vi "RepIntCalc.vi"(8 "SpindleSize":i32, 9 "Look Ahead":i32, 10 "Interrupt Rate":i32=32, 11 "Current Encoder Position":i32) -> (3 "Diff Index":dbl)   [LabVIEW 2010, in "KevLib01.lvlib"]
uses:
  KevLib01.lvlib
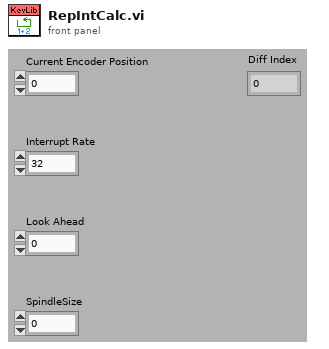
[diagram p1: front panel]
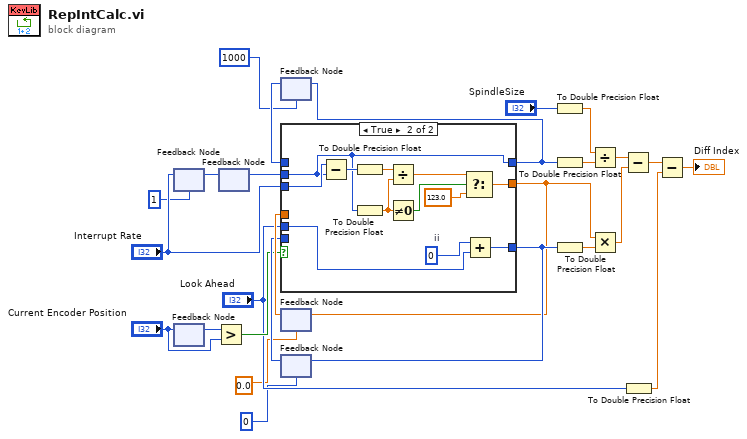
[diagram p0: block diagram]
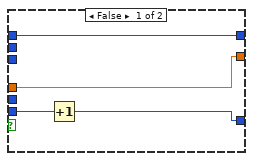
[diagram p2: hidden frame]
diagram:
  n1 = feedback-in #1("Interrupt Rate") -> ()
  n2 = feedback #1(1 ("Interrupt Rate")) -> (w2:i32)
  n3 = feedback-in #2("Current Encoder Position") -> ()
  n4 = feedback #2() -> (w20:i32)  [unwired: 1 out]
  n5 = Greater?(x=w20, y="Current Encoder Position") -> (0:w14:bool)
  n6 = feedback-in #3(w2) -> ()
  n7 = feedback #3() -> (w1:i32)  [unwired: 1 out]
  n8 = feedback #4(1000 ("Interrupt Rate")) -> (w24:i32)
  n9 = feedback #5(0.0 ("f")) -> (w16:dbl)
  n10 = feedback #6(0) -> (w15:i32)
  n11 = case shown="True" w14 {
    tunnel: [w29 w34] -> w19
    tunnel: w15 -> [w30 _]
    tunnel: "Interrupt Rate" -> [_ w41]
    tunnel: w1 -> [_ w39]
    tunnel: [w28 w37] -> w18
    tunnel: w16 -> [w28 _]
    tunnel: [w27 w39] -> w23
    tunnel: w24 -> [w27 _]
    tunnel: "Look Ahead" -> [_ w35]
    frame False {
      n12 = Increment(x=w30) -> (x+1=w29:i32)
    }
    frame True {
      w36 = 0  # ii
      n13 = Subtract(x=w41, y=w39) -> (x-y=w42:i32)
      n14 = To Double Precision Float(number=w42) -> (double precision float=w40:dbl)
      n15 = To Double Precision Float(number=w39) -> (double precision float=w32:dbl)
      n16 = Divide(x=w40, y=w32) -> (x/y=w33:dbl)
      n17 = Not Equal To 0?(x=w32) -> (x != 0?=w31:bool)
      n18 = Select(t=w33, s=w31, f=123.0) -> (s? t:f=w37:dbl)
      n19 = Add(x=w36, y=w35) -> (x+y=w34:i32)
    }
  }
  n20 = feedback-in #4(w23) -> ()
  n21 = feedback-in #5(w18) -> ()
  n22 = feedback-in #6(w19) -> ()
  n23 = To Double Precision Float(number="SpindleSize") -> (double precision float=w11:dbl)
  n24 = To Double Precision Float(number=w23) -> (double precision float=w12:dbl)
  n25 = To Double Precision Float(number=w19) -> (double precision float=w17:dbl)
  n26 = Divide(x=w11, y=w12) -> (x/y=w22:dbl)
  n27 = Multiply(x=w18, y=w17) -> (x*y=w25:dbl)
  n28 = Subtract(x=w22, y=w25) -> (x-y=w10:dbl)
  n29 = To Double Precision Float(number="Look Ahead") -> (double precision float=w9:dbl)
  n30 = Subtract(x=w10, y=w9) -> (x-y=→"Diff Index":dbl)
